vi "LD2018_ブロック崩し_BallSpeed変化.vi"(2 "Speed入力":dbl, 3 "Combo":i32) -> (0 "Speed出力":dbl)   [LabVIEW 2016]
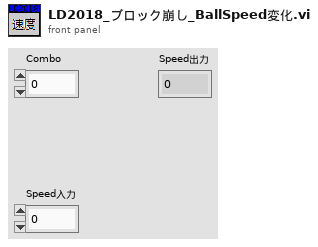
[diagram p1: front panel]
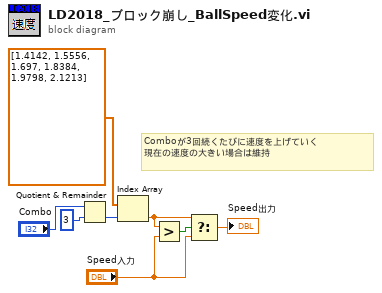
[diagram p0: block diagram]
diagram:
  # "Comboが3回続くたびに速度を上げていく\n現在の速度の大きい場合は維持"
  n1 = Quotient & Remainder(x="Combo", y=3) -> (floor(x/y)=w4:i32)  [unwired: 1 out]
  n2 = Index Array(array=dbl[] [1.4142, 1.5556, 1.697, 1.8384, 1.9798, 2.1213], index=w4) -> (element=w6:dbl)
  n3 = Greater?(x=w6, y="Speed入力") -> (0:w5:bool)
  n4 = Select(t=w6, s=w5, f="Speed入力") -> (s? t:f=→"Speed出力":dbl)
